vi "roi_falls_nicht_gefunden.vi"(4 "Bottom":i32, 6 "Right":i32, 7 "ROI Descriptor in":T1 {"Contours"."Type" items=["No Selection", "Point", "Line", "Rectangle", "Oval", "Polygon", "Freehand Region", "Annulus", "Unused2", "Unused3", "Broken Line", "Freehand Line", "Rotated Rectangle"]}, 9 "Top":i32, 10 "Left":i32, 11 "Boolean":bool) -> (3 "ROI Descriptor out":T1 {"Contours"."Type" items=["No Selection", "Point", "Line", "Rectangle", "Oval", "Polygon", "Freehand Region", "Annulus", "Unused2", "Unused3", "Broken Line", "Freehand Line", "Rotated Rectangle"]})   [LabVIEW 2014]
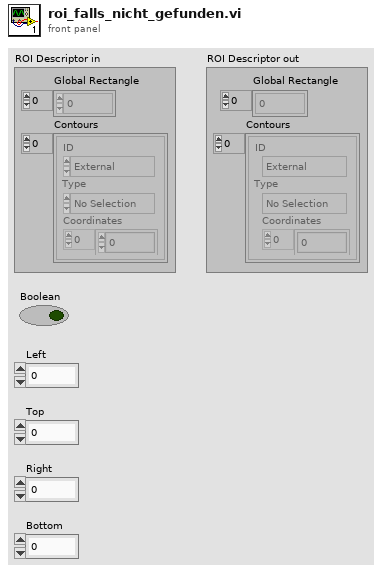
[diagram p1: front panel]
types:
  T1 = typedef "ROI Descriptor" = cluster{"Global Rectangle":i32[], "Contours":cluster{"ID":enum32{"External", "Internal"}, "Type":u32, "Coordinates":i32[]}[]}
  T2 = typedef "IMAQ Rectangle" = cluster{"Left":i32, "Top":i32, "Right":i32, "Bottom":i32, "Rotation":dbl}
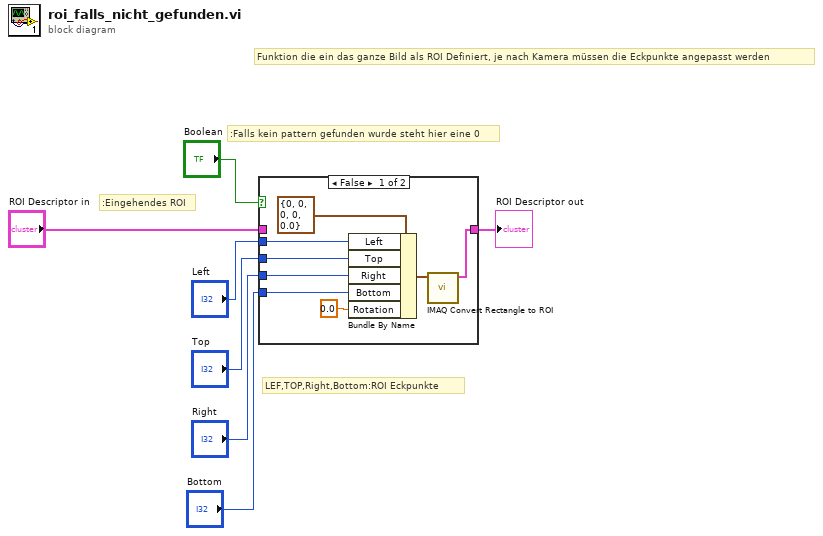
[diagram p0: block diagram]
diagram:
  # "LEF,TOP,Right,Bottom:ROI Eckpunkte"
  # ":Eingehendes ROI"
  # ":Falls kein pattern gefunden wurde steht hier eine 0"
  # "Funktion die ein das ganze Bild als ROI Definiert, je nach Kamera müssen die Eckpunkte angepasst werden"
  n1 = case shown="False" "Boolean" {
    tunnel: [w12 w16] -> w3
    tunnel: "ROI Descriptor in" -> [_ w16]
    tunnel: "Left" -> [w11 _]
    tunnel: "Top" -> [w10 _]
    tunnel: "Right" -> [w9 _]
    tunnel: "Bottom" -> [w8 _]
    frame False {
      n2 = Bundle By Name(cluster=T2 {"Left"=0, "Top"=0, "Right"=0, "Bottom"=0, "Rotation"=0.0} ("Rectangle"), "Left"=w11, "Top"=w10, "Right"=w9, "Bottom"=w8, "Rotation"=0.0) -> (w13:T2)
      n3 = call "IMAQ Convert Rectangle to ROI"("Rectangle"=w13) -> ("ROI Descriptor"=w12:T1)  [unwired: 8 in, 1 out]
    }
    frame True {
    }
  }
  "ROI Descriptor out" <- w3
